vi "AMAFPP Pre-Install Custom Action.vi"(10 "Variant":variant) -> (0 "error out":errorcluster)   [LabVIEW 2023]
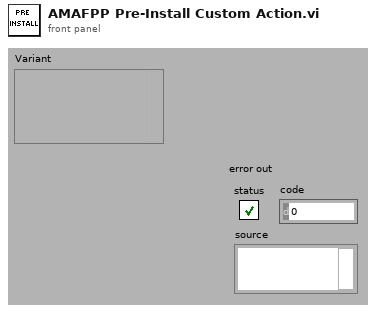
[diagram p1: front panel]
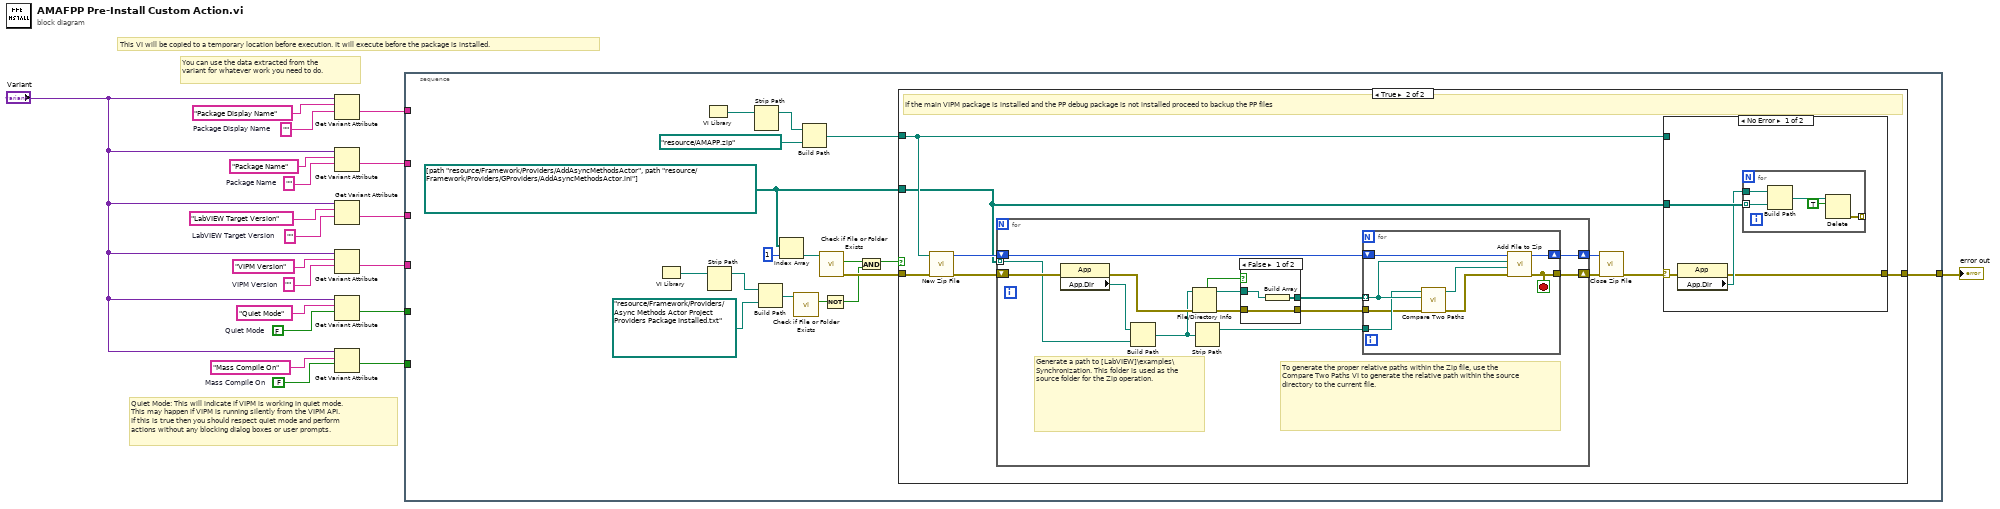
[diagram p0: block diagram]
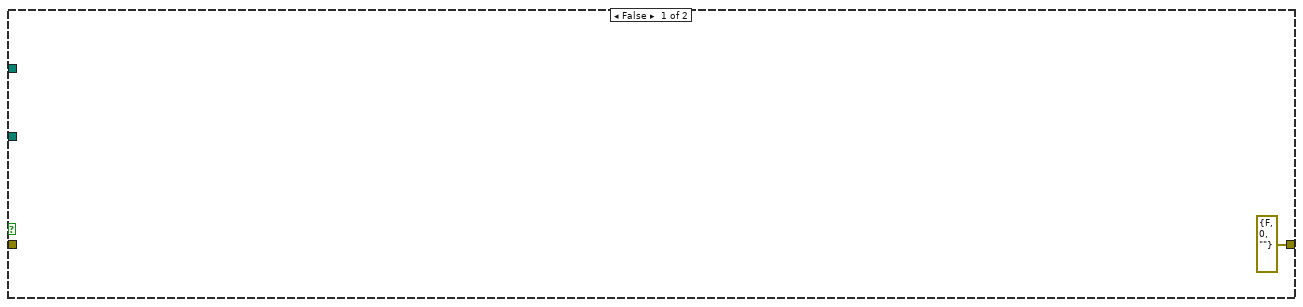
[diagram p2: hidden frame]
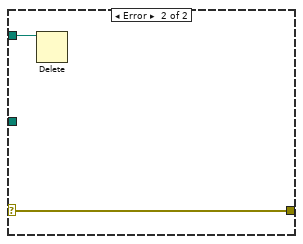
[diagram p3: hidden frame]
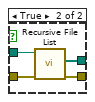
[diagram p4: hidden frame]
diagram:
  w2 = FALSE  # Mass Compile On
  w4 = ""  # Package Display Name
  w11 = FALSE  # Quiet Mode
  w14 = ""  # VIPM Version
  w16 = ""  # LabVIEW Target Version
  w18 = ""  # Package Name
  # "You can use the data extracted from the variant for whatever work you need to do."
  # "Quiet Mode: This will indicate if VIPM is working in quiet mode.\nThis may happen if VIPM is running silently from the VIPM API.\nIf this is true then you should respect quiet mode and perform\nactions without any blocking dialog boxes or user prompts."
  # "This VI will be copied to a temporary location before execution. It will execute before the package is installed."
  n1 = Get Variant Attribute(Variant="Variant", name="Package Display Name", default value (empty Variant)=w4) -> (value=w10:string)  [unwired: 1 in, 3 out]
  n2 = Get Variant Attribute(Variant="Variant", name="Package Name", default value (empty Variant)=w18) -> (value=w9:string)  [unwired: 1 in, 3 out]
  n3 = Get Variant Attribute(Variant="Variant", name="LabVIEW Target Version", default value (empty Variant)=w16) -> (value=w8:string)  [unwired: 1 in, 3 out]
  n4 = Get Variant Attribute(Variant="Variant", name="VIPM Version", default value (empty Variant)=w14) -> (value=w7:string)  [unwired: 1 in, 3 out]
  n5 = Get Variant Attribute(Variant="Variant", name="Quiet Mode", default value (empty Variant)=w11) -> (value=w6:bool)  [unwired: 1 in, 3 out]
  n6 = Get Variant Attribute(Variant="Variant", name="Mass Compile On", default value (empty Variant)=w2) -> (value=w5:bool)  [unwired: 1 in, 3 out]
  n7 = stacked-sequence {
    tunnel: w10 -> [_]
    tunnel: w9 -> [_]
    tunnel: w8 -> [_]
    tunnel: w7 -> [_]
    tunnel: w6 -> [_]
    tunnel: w5 -> [_]
    tunnel: [w37] -> w1
    frame #0 {
      w30 = path[] [path "resource/Framework/Providers/AddAsyncMethodsActor", path "resource/Framework/Providers/GProviders/AddAsyncMethodsActor.ini"]
      n8 = VI Library() -> (path=w27:path)
      n9 = VI Library() -> (path=w35:path)
      n10 = Strip Path(path=w27) -> (stripped path=w25:path)  [unwired: 1 out]
      n11 = Strip Path(path=w35) -> (stripped path=w33:path)  [unwired: 1 out]
      n12 = Build Path(base path=w25, name or relative path=path "resource/Framework/Providers/Async Methods Actor Project Providers Package Installed.txt") -> (appended path=w24:path)
      n13 = Index Array(array=w30, index=1) -> (element=w32:path)
      n14 = call <vilib>:"Check if File or Folder Exists.vi"("path"=w24) -> ("file or folder exists?"=w23:bool)  [unwired: 8 in, 2 out]
      n15 = Build Path(base path=w33, name or relative path=path "resource/AMAPP.zip") -> (appended path=w36:path)
      n16 = call <vilib>:"Check if File or Folder Exists.vi"("path"=w32) -> ("error out"=w28:errorcluster, "file or folder exists?"=w29:bool)  [unwired: 8 in, 1 out]
      n17 = Not(x=w23) -> (.not. x?=w21:bool)
      n18 = And(x=w29, y=w21) -> (x .and. y?=w22:bool)
      n19 = case shown="True" w22 {
        tunnel: [errorcluster {"status"=FALSE, "code"=0, "source"=""} ("error IO") w47] -> w37
        tunnel: w36 -> [_ w46]
        tunnel: w30 -> [_ w40]
        tunnel: w28 -> [_ w39]
        frame False {
        }
        frame True {
          # "If the main VIPM package is installed and the PP debug package is not installed proceed to backup the PP files"
          n20 = call <vilib>:"New Zip File.vi"("error in (no error)"=w39, "target"=w46) -> ("error out"=w42:errorcluster, "zip file out"=w41:i64)  [unwired: 1 in, 3 out]
          n21 = for {
            shift-right: [w71] -> w43
            shift-left: w42 -> [w72]
            tunnel: w40 -> [w70] mode=indexing
            shift-right: [w59] -> w44
            shift-left: w41 -> [w69]
            # "Generate a path to [LabVIEW]\\examples\\Synchronization. This folder is used as the source folder for the Zip operation."
            # "To generate the proper relative paths within the Zip file, use the Compare Two Paths VI to generate the relative path within the source directory to the current file."
            n22 = property class="App"(error in=w72) -> (error out=w68:errorcluster, "App.Dir"=w61:path)  [unwired: 1 in, 1 out]
            n23 = Build Path(base path=w61, name or relative path=w70) -> (appended path=w64:path)
            n24 = File/Directory Info(path=w64, error in=w68) -> (path out=w65:path, directory=w66:bool, error out=w63:errorcluster)  [unwired: 4 out]
            n25 = Strip Path(path=w64) -> (stripped path=w67:path)  [unwired: 1 out]
            n26 = case shown="False" w66 {
              tunnel: [w73 w79] -> w60
              tunnel: [w75 w78] -> w62
              tunnel: w63 -> [w75 w77]
              tunnel: w65 -> [w74 w76]
              frame False {
                n27 = Build Array(w74) -> (w73:path[])
              }
              frame True {
                n28 = call <vilib>:"Recursive File List.vi"("error in (no error)"=w77, "Folder Path"=w76) -> ("error out"=w78:errorcluster, "All Files in Dir"=w79:path[])  [unwired: 5 in, 3 out]
              }
            }
            n29 = for {
              tunnel: w60 -> [w84] mode=indexing
              tunnel: w62 -> [w81]
              tunnel: [w85] -> w71
              shift-right: [w86] -> w59
              shift-left: w69 -> [w87]
              tunnel: w67 -> [w83]
              stop <- w85 stop-if-true
              n30 = call <vilib>:"Compare Two Paths.vi"("error in (no error)"=w81, "Path 2"=w84, "Path 1"=w83) -> ("error out"=w80:errorcluster, "Relative Path from 1 to 2"=w82:path)  [unwired: 5 in, 2 out]
              n31 = call <vilib>:"Add File to Zip.vi"("error in (no error)"=w80, "destination path in zip"=w82, "source file path"=w84, "zip file in"=w87) -> ("error out"=w85:errorcluster, "zip file out"=w86:i64)  [unwired: 6 out]
            }
          }
          n32 = call <vilib>:"Close Zip File.vi"("error in (no error)"=w43, "zip file in"=w44) -> ("error out"=w45:errorcluster)  [unwired: 1 in, 4 out]
          n33 = case shown="No Error" w45 {
            selector: w45 -> [w51 w58]
            tunnel: [w48 w58] -> w47
            tunnel: w46 -> [_ w57]
            tunnel: w40 -> [w50 _]
            frame No Error {
              n34 = property class="App"(error in=w51) -> (error out=w48:errorcluster, "App.Dir"=w49:path)  [unwired: 1 in, 1 out]
              n35 = for {
                tunnel: w50 -> [w56] mode=indexing
                tunnel: w49 -> [w54]
                tunnel: [w53] -> _ mode=indexing
                n36 = Build Path(base path=w54, name or relative path=w56) -> (appended path=w55:path)
                n37 = Delete(path (use dialog)=w55, entire hierarchy (F)=TRUE) -> (error out=w53:errorcluster)  [unwired: 3 in, 2 out]
              }
            }
            frame Error {
              n38 = Delete(path (use dialog)=w57) -> ()  [unwired: 4 in, 3 out]
            }
          }
        }
      }
    }
  }
  "error out" <- w1
